vi "RestartProbeCycle.vi"(9 "WaferAlignment":T1, 10 "Position":i32[](array[numeric]), 11 "Array":T2(array[cluster])) -> (3 "Numeric":i32)   [LabVIEW 2020]
uses:
  WaferAlignmentType.ctl
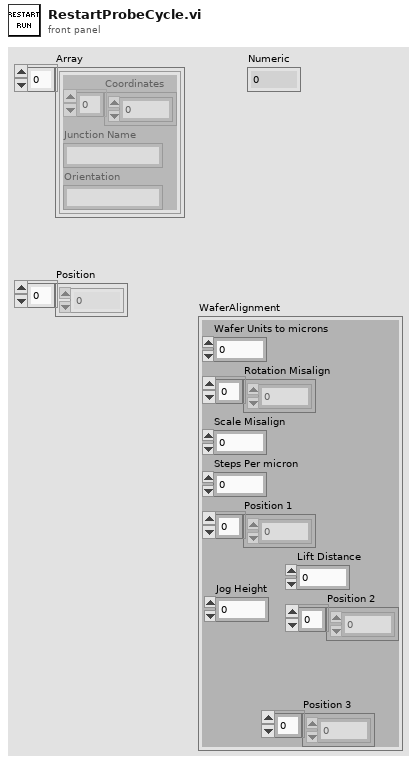
[diagram p1: front panel]
types:
  T1 = typedef "WaferAlignmentType.ctl" = cluster{"Wafer Units to microns":dbl, "Rotation Misalign":dbl[], "Scale Misalign":dbl, "Steps Per micron":dbl, "Position 1":i32[], "Position 2":i32[], "Lift Distance":i32, "Position 3":i32[], "Jog Height":i32}
  T2 = cluster{"Coordinates":dbl[], "Junction Name":string, "Orientation":string}[]
  T3 = cluster{"Coordinates":dbl[], "Junction Name":string, "Orientation":string}
  T4 = enum16{"Left Button", "Center Button", "Right Button", "Window Close"}
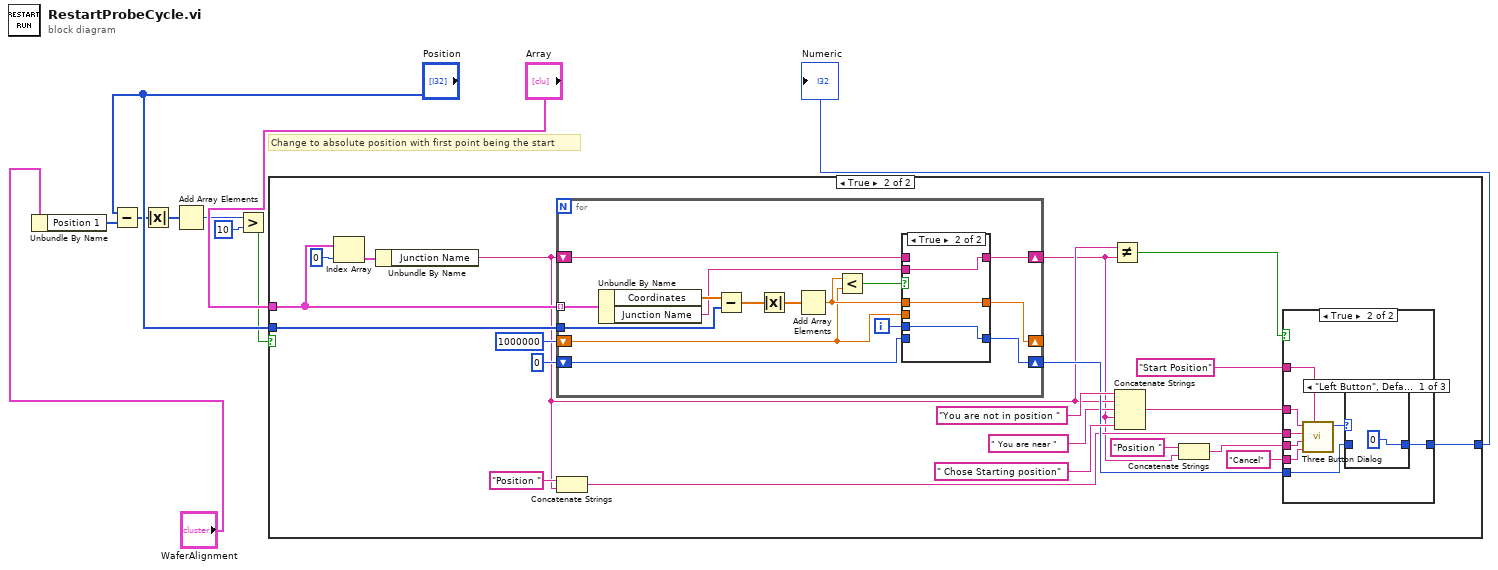
[diagram p0: block diagram]
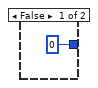
[diagram p2: hidden frame]
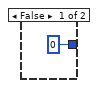
[diagram p3: hidden frame]
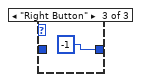
[diagram p5: hidden frame]
diagram:
  # "Change to absolute position with first point being the start"
  n1 = Unbundle By Name("WaferAlignment") -> ("Position 1"=w9:i32[])
  n2 = Subtract(x="Position", y=w9) -> (x-y=w2:i32[])
  n3 = Absolute Value(x=w2) -> (abs(x)=w3:i32[])
  n4 = Add Array Elements(numeric array=w3) -> (sum=w4:i32)
  n5 = Greater?(x=w4, y=10) -> (0:w6:bool)
  n6 = case shown="True" w6 {
    tunnel: [0 w25] -> w7
    tunnel: "Array" -> [_ w22]
    tunnel: "Position" -> [_ w15]
    frame False {
    }
    frame True {
      n7 = Index Array(array=w22, index=0) -> (element=w31:T3)
      n8 = Unbundle By Name(w31) -> ("Junction Name"=w14:string)
      n9 = for {
        tunnel: w22 -> [w57] mode=indexing
        tunnel: w15 -> [w55]
        shift-right: [w49] -> w20
        shift-left: 0 -> [w48]
        shift-right: [w50] -> w13
        shift-left: w14 -> [w51]
        shift-right: [w47] -> _
        shift-left: 1000000 -> [w45]
        i -> [w52]
        n10 = Unbundle By Name(w57) -> ("Coordinates"=w56:dbl[], "Junction Name"=w54:string)
        n11 = Subtract(x=w56, y=w55) -> (x-y=w59:dbl[])
        n12 = Absolute Value(x=w59) -> (abs(x)=w58:dbl[])
        n13 = Add Array Elements(numeric array=w58) -> (sum=w46:dbl)
        n14 = Less?(x=w46, y=w45) -> (x < y?=w53:bool)
        n15 = case shown="True" w53 {
          tunnel: w54 -> [_ w65]
          tunnel: w51 -> [w62 _]
          tunnel: [w62 w65] -> w50
          tunnel: w52 -> [_ w64]
          tunnel: [w61 w64] -> w49
          tunnel: w48 -> [w61 _]
          tunnel: w45 -> [w60 _]
          tunnel: [w60 w63] -> w47
          tunnel: w46 -> [_ w63]
          frame False {
          }
          frame True {
          }
        }
      }
      n16 = Concatenate Strings("Position " ("Left Button Text (\"Yes\")"), w14) -> (w17:string)
      n17 = Not Equal?(x=w14, y=w13) -> (x != y?=w12:bool)
      n18 = Concatenate Strings("You are not in position " ("message"), w14, " You are near " ("string"), w13, " Chose Starting position" ("string")) -> (w28:string)
      n19 = Concatenate Strings("Position " ("string"), w13) -> (w27:string)
      n20 = case shown="True" w12 {
        tunnel: "Cancel" ("Right Button Text (\"Cancel\")") -> [_ w41]
        tunnel: w28 -> [_ w40]
        tunnel: w27 -> [_ w39]
        tunnel: [0 w38] -> w25
        tunnel: "Start Position" ("Window Title (\"\")") -> [_ w36]
        tunnel: w20 -> [_ w35]
        tunnel: w17 -> [_ w34]
        frame False {
        }
        frame True {
          n21 = call <vilib>:"Three Button Dialog.vi"("Window Title (\"\")"=w36, "Right Button Text (\"Cancel\")"=w41, "Center Button Text (\"No\")"=w39, "Left Button Text (\"Yes\")"=w34, "message"=w40) -> ("Which Button?"=w37:T4)  [unwired: 6 in]
          n22 = case shown="\"Left Button\", Default" w37 {
            tunnel: [0 w43 -1] -> w38
            tunnel: w35 -> [_ w43 _]
            frame "Left Button", Default {
            }
            frame "Center Button" {
            }
            frame "Right Button" {
            }
          }
        }
      }
    }
  }
  "Numeric" <- w7
